vi "Read zxd time.vi"(8 "error in (no error)":errorcluster caption="에러 입력(에러 없음)", 11 "Auto Tracking Wave 입력":refnum<class "Auto Track Wave.lvclass">) -> (0 "error out":errorcluster caption="에러 출력", 2 "zxd time":u8=6, 3 "Auto Tracking Wave 출력":refnum<class "Auto Track Wave.lvclass">)   [LabVIEW 2020, in "Auto Track Wave.lvclass"]
uses:
  Auto Track Wave.lvclass
  Auto Track Wave.lvclass/Auto Track Wave.ctl
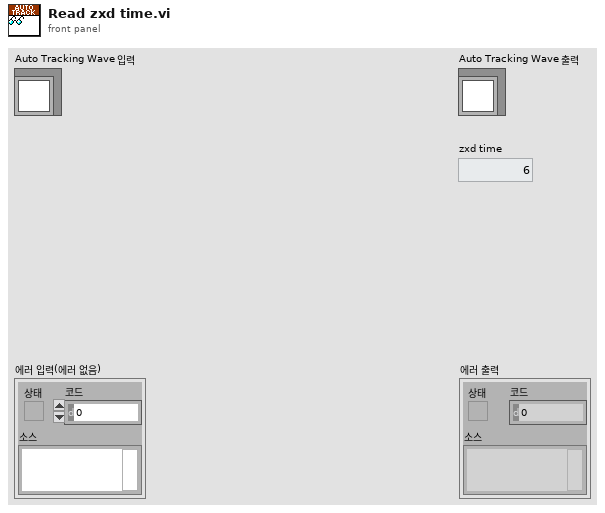
[diagram p1: front panel]
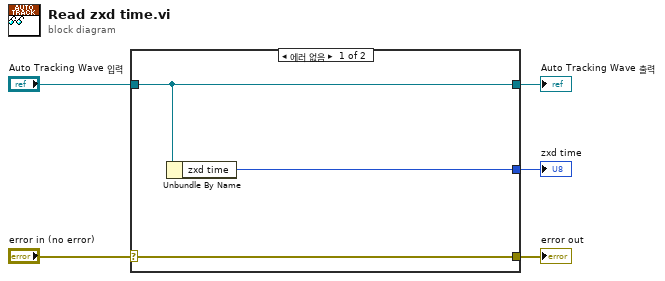
[diagram p0: block diagram]
diagram:
  n1 = case shown="에러 없음" "error in (no error)" {
    selector: "error in (no error)" -> [w8 w9]
    tunnel: [w8 w9] -> w4
    tunnel: [w7 w10] -> w2
    tunnel: "Auto Tracking Wave 입력" -> [w7 w10]
    tunnel: [w6 _] -> w1
    frame No Error {
      n2 = Unbundle By Name(w7) -> ("zxd time"=w6:u8)
    }
    frame Error {
    }
  }
  "error out" <- w4
  "Auto Tracking Wave 출력" <- w2
  "zxd time" <- w1
